vi "configure accesspoint.vi"(9 "radio2_pipe_count":u8, 10 "radio1_pipe_count":u8, 11 "ap_handle":u32) -> (2 "function return":i32, 3 "ap_handle out":u32)   [LabVIEW 2019, in "apdm.lvlib"]
doc: "APDM_EXPORT int apdm_configure_accesspoint(apdm_ap_handle_t ap_handle, const uint8_t radio1_pipe_count, const uint8_t radio2_pipe_count);"
uses:
  apdm.lvlib
  Lee Lab/CP FES Walking 2018/Code/Working/LabVIEW/apdm.dll
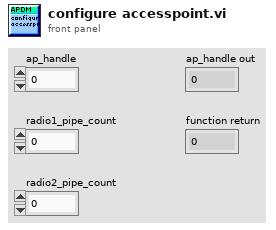
[diagram p1: front panel]
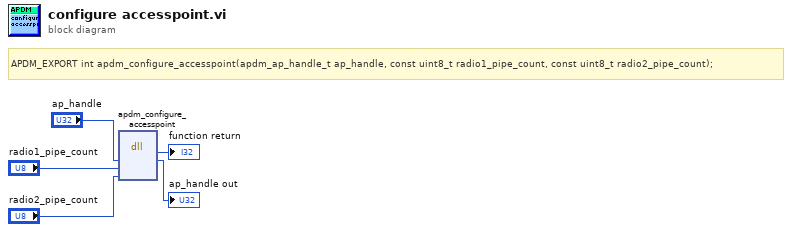
[diagram p0: block diagram]
diagram:
  # "APDM_EXPORT int apdm_configure_accesspoint(apdm_ap_handle_t ap_handle, const uint8_t radio1_pipe_count, const uint8_t radio2_pipe_count);"
  n1 = dll-call lib="C:/Users/jfalesi/Dropbox/Lee Lab/CP FES Walking 2018/Code/Working/LabVIEW/apdm.*" fn="apdm_configure_accesspoint"("ap_handle"="ap_handle", "radio1_pipe_count"="radio1_pipe_count", "radio2_pipe_count"="radio2_pipe_count") -> (→"function return":i32, "ap_handle"=→"ap_handle out":u32)  [unwired: 5 in, 2 out]
